vi "Main.vi"() -> ()   [LabVIEW 2020]
doc: "Use this template to build a simple state machine design pattern. Each state executes code and determines which state to transition to."
uses:
  controls/Data.ctl
  Control 1.ctl
  <vilib>/numeric/Random Number (Range) I64.vi
  <vilib>/numeric/sub_Random U32.vi
panel:
  out "Genius":u32[](array[colorbox])
  in  "Cluster":T1
  out "Genius Display":u32(colorbox)
  out "history":i64
  out "Colours":u32[](array[colorbox])
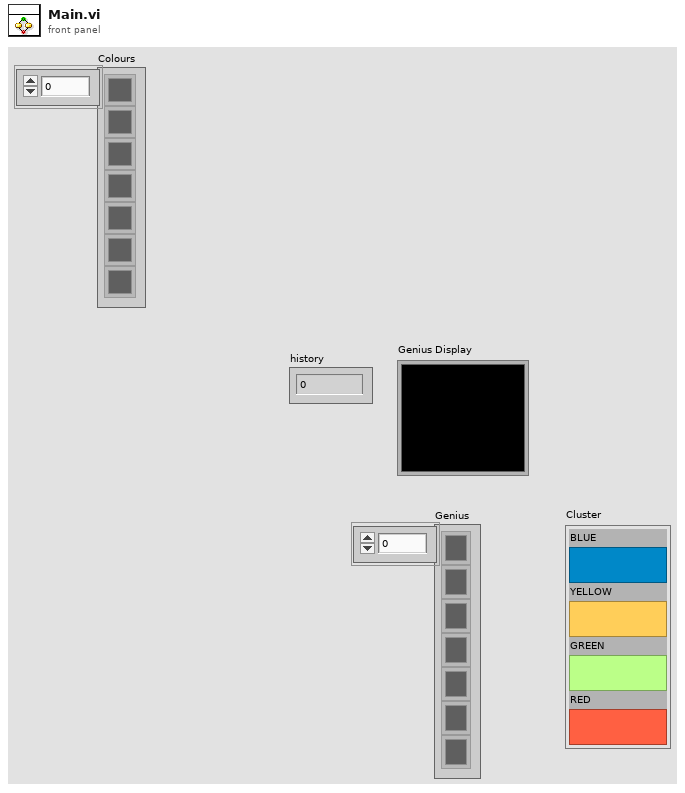
[diagram p1: front panel]
types:
  T1 = cluster{"BLUE":bool, "YELLOW":bool, "GREEN":bool, "RED":bool}
  T2 = typedef "Control 1.ctl" = enum32{"Play", "Initialise", "Create Colours", "Show colours sequence", "Wait for event", "array size", "Press colours sequence", "Compare colours", "Success ", "Failure", "Exit"}
  T3 = typedef "Data.ctl" = cluster{"Colours":i64[], "history ":i64[], "Wait time(ms)":u64, "String":string, "picked color":i64, "User's turn":i64}
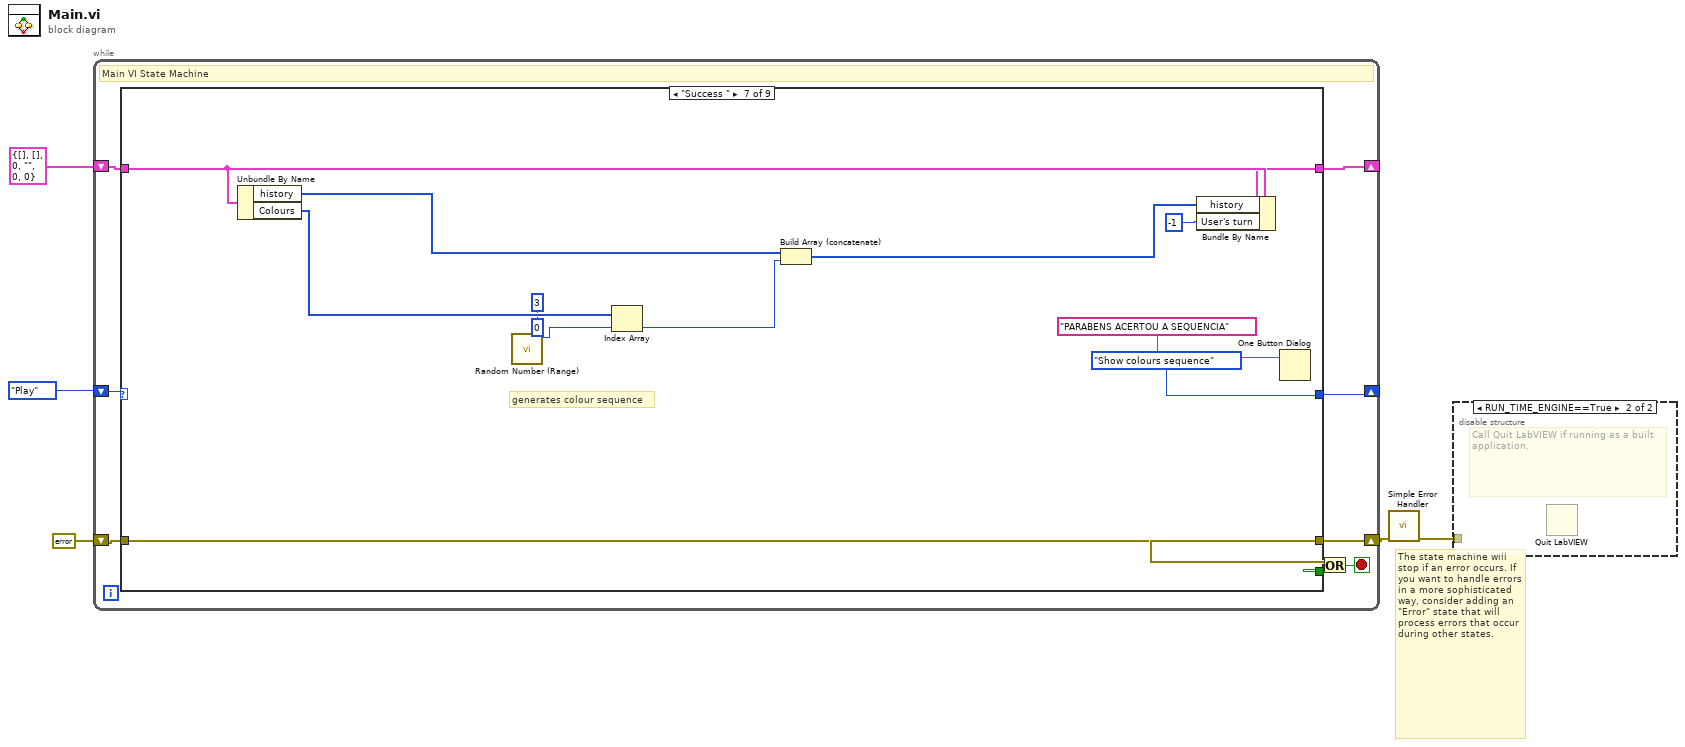
[diagram p0: block diagram]
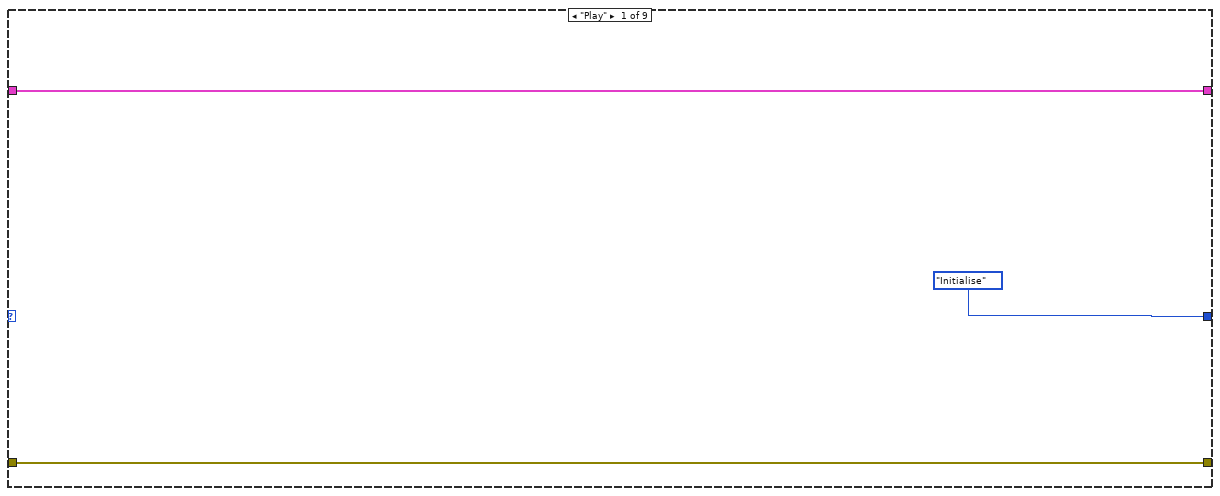
[diagram p3: hidden frame]
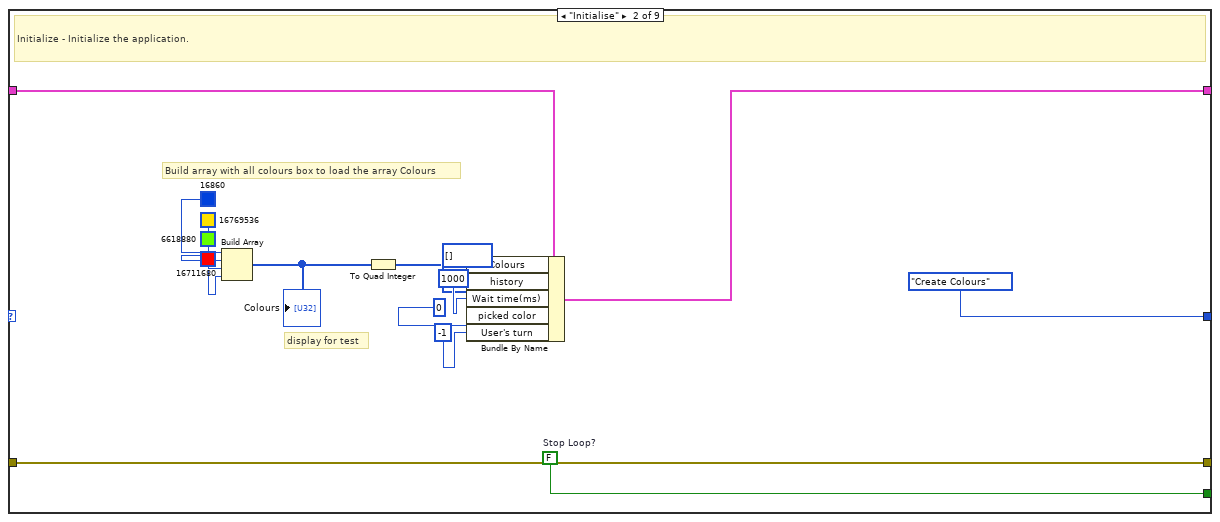
[diagram p4: hidden frame]
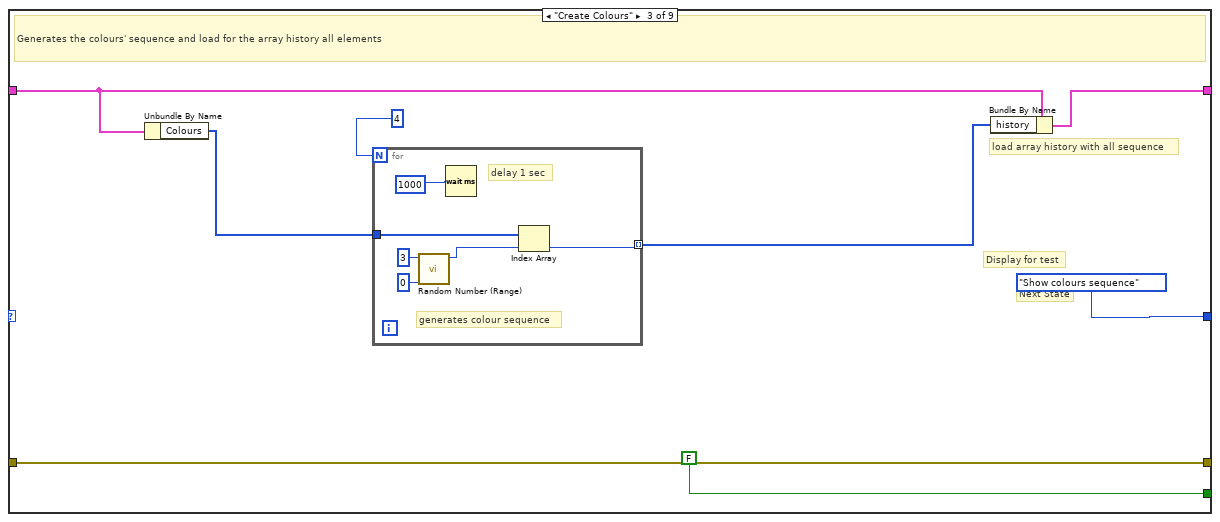
[diagram p5: hidden frame]
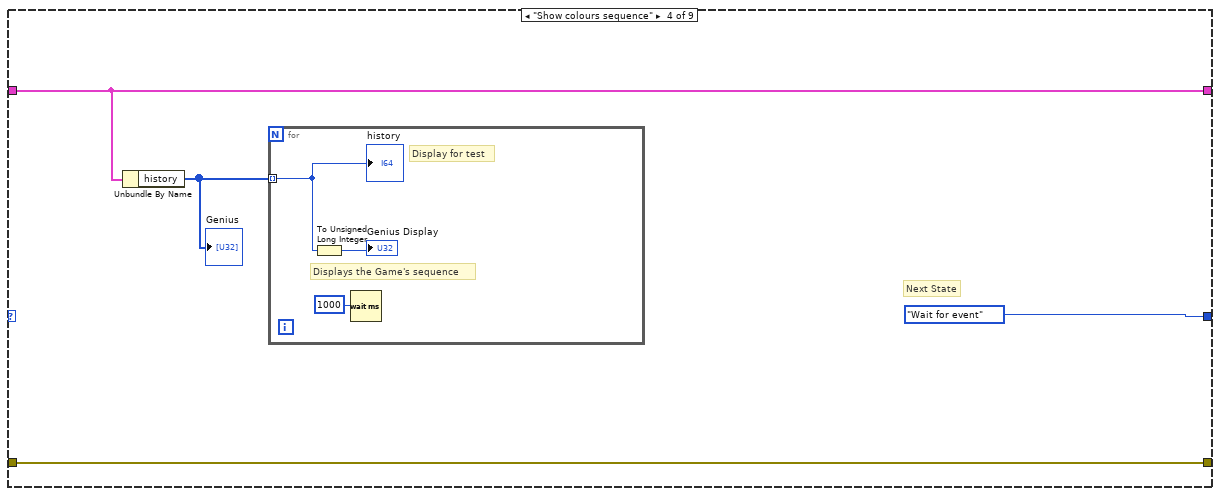
[diagram p6: hidden frame]
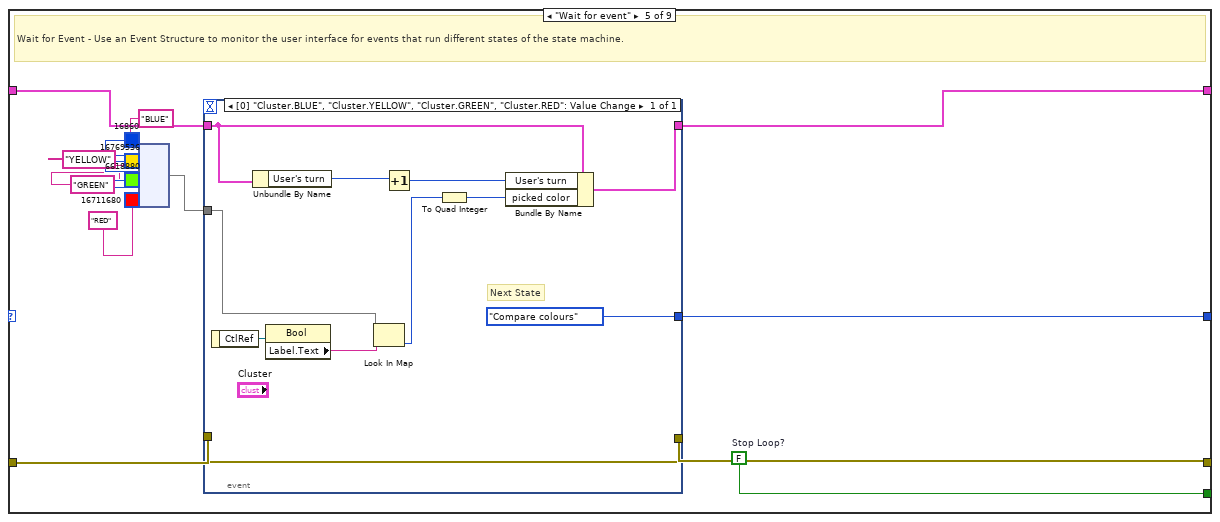
[diagram p7: hidden frame]
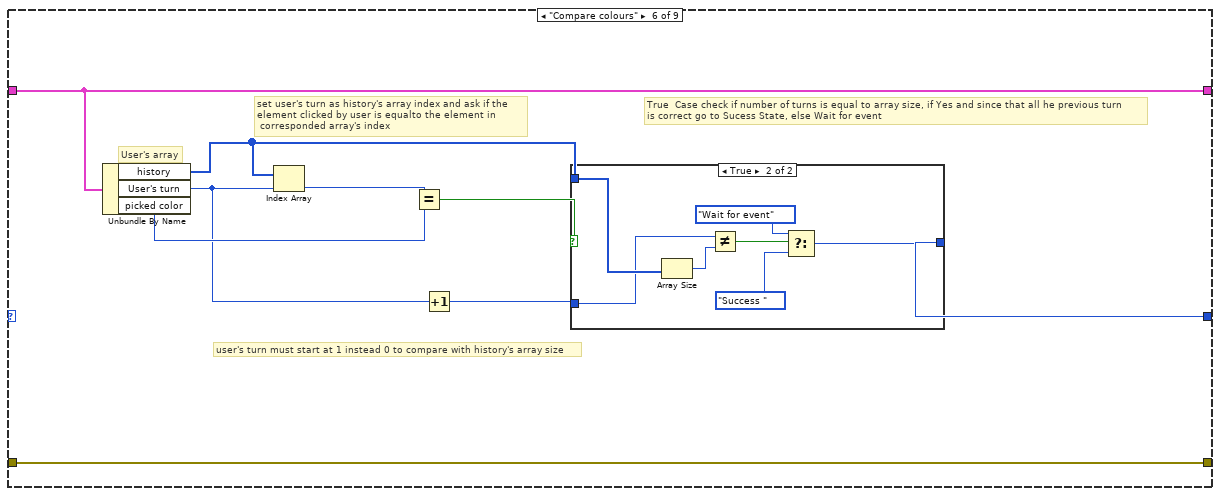
[diagram p8: hidden frame]
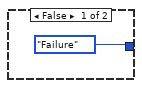
[diagram p9: hidden frame]
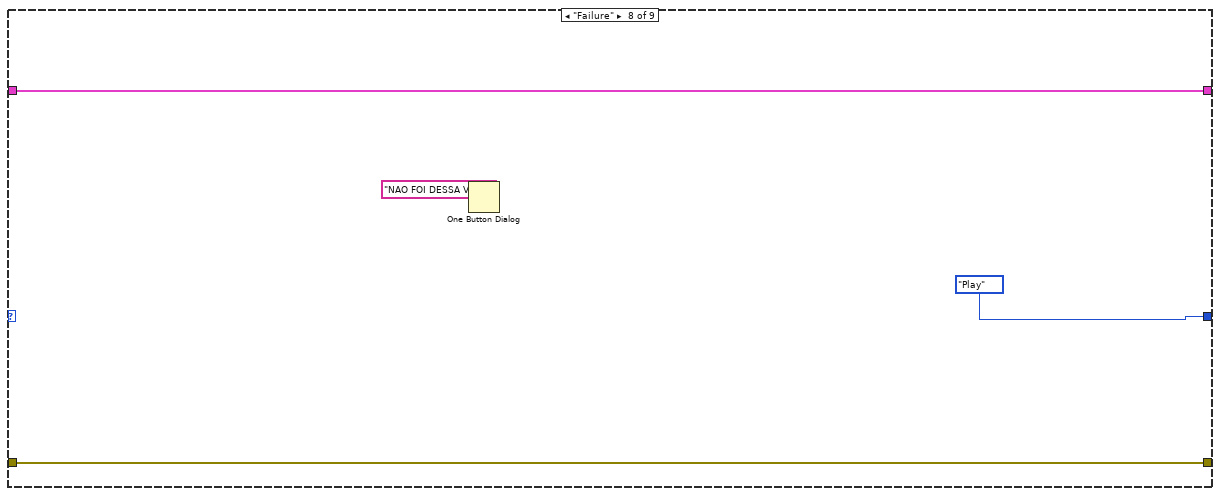
[diagram p10: hidden frame]
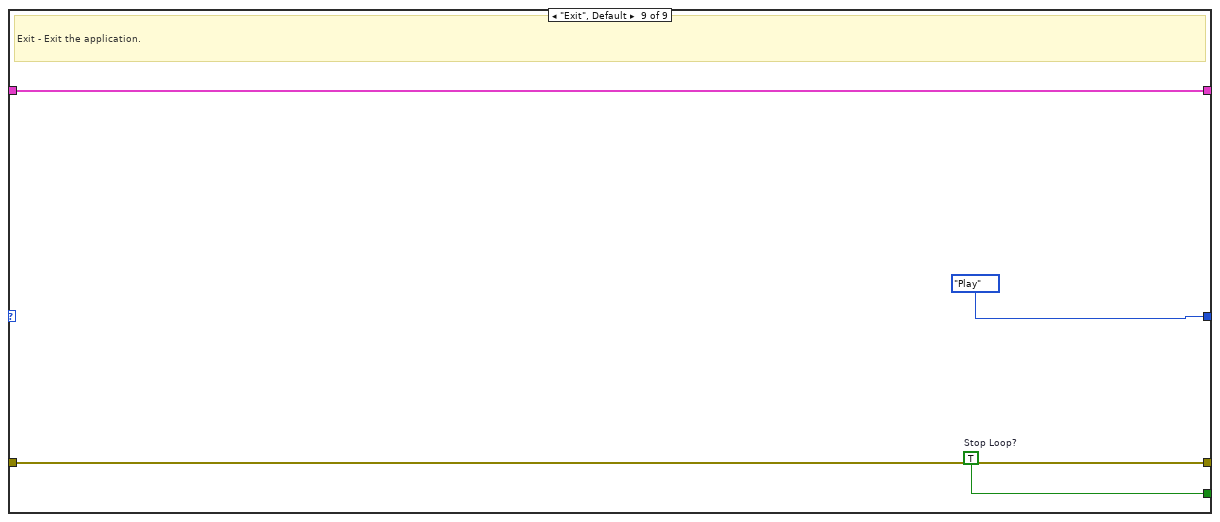
[diagram p11: hidden frame]
diagram:
  # "The state machine will stop if an error occurs. If you want to handle errors in a more sophisticated way, consider adding an \"Error\" state that will process errors that occur during other states."
  n1 = while {
    shift-right: [w12] -> _
    shift-left: T3 {"Colours"=[], "history "=[], "Wait time(ms)"=0, "String"="", "picked color"=0, "User's turn"=0} ("Data") -> [w13]
    shift-right: [w8] -> w3
    shift-left: errorcluster {"status"=FALSE, "code"=0, "source"=""} ("error constant") -> [w11]
    shift-right: [w6] -> _
    shift-left: Control_1."Play" -> [w7]
    stop <- w9 stop-if-true
    # "Main VI State Machine"
    n2 = case shown="\"Success \"" w7 {
      tunnel: [Control_1."Initialise" Control_1."Create Colours" Control_1."Show colours sequence" Control_1."Wait for event" w54 w81 Control_1."Show colours sequence" Control_1."Play" Control_1."Play"] -> w6
      tunnel: [_ w31 FALSE ("Stop Loop?") _ w67 _ _ _ w115] -> w10
      tunnel: w13 -> [w16 w25 w36 w48 w66 w86 w101 w112 w116]
      tunnel: [w16 w24 w35 w48 w53 w86 w97 w112 w116] -> w12
      tunnel: w11 -> [w15 w30 w38 w49 w65 w87 w108 w111 w114]
      tunnel: [w15 w30 w38 w49 w64 w87 w108 w111 w114] -> w8
      frame "Play" {
      }
      frame "Initialise" {
        w31 = FALSE  # Stop Loop?
        # "display for test"
        # "Build array with all colours box to load the array Colours"
        # "Initialize - Initialize the application."
        n3 = Build Array(u32 16860, u32 16769536, u32 6618880, u32 16711680) -> (w19:u32[])
        "Colours" <- w19
        n4 = To Quad Integer(1:w19) -> (0:w18:i64[])
        n5 = Bundle By Name(cluster=w25, "Colours"=w18, "history"=i64[] [], "Wait time(ms)"=u64 1000, "picked color"=u64 0, "User's turn"=i64 -1) -> (w24:T3)
      }
      frame "Create Colours" {
        # "Display for test"
        # "Next State"
        # "load array history with all sequence"
        # "Generates the colours' sequence and load for the array history all elements"
        n6 = Unbundle By Name(w36) -> ("Colours"=w32:i64[])
        n7 = for {
          N: 4 -> [_]
          tunnel: w32 -> [w43]
          tunnel: [w45] -> w34 mode=indexing
          # "delay 1 sec"
          # "generates colour sequence"
          n8 = call-poly <vilib>:"Random Number (Range).vi"("lower bound (-100)"=i64 0, "upper bound (100)"=i64 3) -> ("number"=w40:i64)  [unwired: 9 in]
          n9 = Wait (ms)(milliseconds to wait=u32 1000 ("millisecond timer value")) -> ()  [unwired: 1 out]
          n10 = Index Array(array=w43, index=w40) -> (element=w45:i64)
        }
        n11 = Bundle By Name(cluster=w36, "history"=w34) -> (w35:T3)
      }
      frame "Show colours sequence" {
        # "Next State"
        n12 = Unbundle By Name(w48) -> ("history"=w46:i64[])
        "Genius" <- w46
        n13 = for {
          tunnel: w46 -> [w50] mode=indexing
          # "Display for test"
          # "Displays the Game's sequence"
          n14 = To Unsigned Long Integer(number=w50) -> (unsigned 32bit integer=→"Genius Display":u32)
          n15 = Wait (ms)(milliseconds to wait=u32 1000 ("millisecond timer value")) -> ()  [unwired: 1 out]
          "history" <- w50
        }
      }
      frame "Wait for event" {
        w67 = FALSE  # Stop Loop?
        # "Wait for Event - Use an Event Structure to monitor the user interface for events that run different states of the state machine."
        n16 = node("BLUE" ("key"), u32 16860, "YELLOW" ("key"), u32 16769536, "GREEN" ("key"), u32 6618880, "RED" ("key"), u32 16711680) -> (w55:map{string, u32})
        n17 = event shown="[0] \"Cluster.BLUE\", \"Cluster.YELLOW\", \"Cluster.GREEN\", \"Cluster.RED\": Value Change" {
          selector: _ -> [_]
          dyn-events: _ -> [_]
          timeout: _ -> [_]
          tunnel: w66 -> [w73]
          tunnel: w65 -> [w78]
          tunnel: [w78] -> w64
          tunnel: w55 -> [w75]
          tunnel: [Control_1."Compare colours" ("f")] -> w54
          tunnel: [w72] -> w53
          event "Cluster.BLUE", "Cluster.YELLOW", "Cluster.GREEN", "Cluster.RED": Value Change {
            # "Next State"
            n18 = event-data() -> ("CtlRef"=w77:refnum<vi>)  [unwired: 1 in]
            n19 = Unbundle By Name(w73) -> ("User's turn"=w71:i64)
            n20 = property class="Bool"(reference=w77) -> ("Label.Text"=w76:string)  [unwired: 1 in, 2 out]
            n21 = Look In Map(map=w75, key=w76) -> (value=w69:u32)  [unwired: 1 in, 1 out]
            n22 = Increment(x=w71) -> (x+1=w70:i64)
            n23 = To Quad Integer(1:w69) -> (0:w68:i64)
            n24 = Bundle By Name(cluster=w73, "User's turn"=w70, "picked color"=w68) -> (w72:T3)
          }
        }
      }
      frame "Compare colours" {
        # "True  Case check if number of turns is equal to array size, if Yes and since that all he previous turn\nis correct go to Sucess State, else Wait for event"
        # "set user's turn as history's array index and ask if the \nelement clicked by user is equalto the element in\n corresponded array's index"
        # "user's turn must start at 1 instead 0 to compare with history's array size"
        # "User's array"
        n25 = Unbundle By Name(w86) -> ("history"=w82:i64[], "User's turn"=w79:i64, "picked color"=w85:i64)
        n26 = Index Array(array=w82, index=w79) -> (element=w84:i64)
        n27 = Equal?(x=w84, y=w85) -> (x = y?=w83:bool)
        n28 = Increment(x=w79) -> (x+1=w80:i64)
        n29 = case shown="True" w83 {
          tunnel: w82 -> [_ w95]
          tunnel: [Control_1."Failure" w91] -> w81
          tunnel: w80 -> [_ w89]
          frame False {
          }
          frame True {
            n30 = Array Size(array=w95) -> (size(s)=w90:i32)
            n31 = Not Equal?(x=w89, y=w90) -> (x != y?=w94:bool)
            n32 = Select(t=Control_1."Wait for event", s=w94, f=Control_1."Success ") -> (s? t:f=w91:T2)
          }
        }
      }
      frame "Success " {
        # "generates colour sequence"
        n33 = Unbundle By Name(w101) -> ("history"=w99:i64[], "Colours"=w105:i64[])
        n34 = call-poly <vilib>:"Random Number (Range).vi"("lower bound (-100)"=i64 0, "upper bound (100)"=i64 3) -> ("number"=w102:i64)  [unwired: 9 in]
        n35 = Index Array(array=w105, index=w102) -> (element=w100:i64)
        n36 = Build Array (concatenate)(w99, w100) -> (w98:i64[])
        n37 = Bundle By Name(cluster=w101, "history"=w98, "User's turn"=i64 -1) -> (w97:T3)
        n38 = One Button Dialog(message="PARABENS ACERTOU A SEQUENCIA") -> ()  [unwired: 1 in, 1 out]
      }
      frame "Failure" {
        n39 = One Button Dialog(message="NAO FOI DESSA VEZ") -> ()  [unwired: 1 in, 1 out]
      }
      frame "Exit", Default {
        w115 = TRUE  # Stop Loop?
        # "Exit - Exit the application."
      }
    }
    n40 = Or(x=w8, y=w10) -> (x .or. y?=w9:bool)
  }
  n41 = call <vilib>:"Simple Error Handler.vi"("error in (no error)"=w3) -> ("error out"=w2:errorcluster)  [unwired: 4 in, 4 out]
  n42 = disable-structure shown="RUN_TIME_ENGINE==True" {
    disable-tunnel: w2 -> [_ _]
    frame condition #0 (active) {
    }
    frame condition #1 {
      # "Call Quit LabVIEW if running as a built application."
      n43 = Quit LabVIEW() -> ()  [unwired: 1 in]
    }
  }
